vi "Create.vi"(8 "error in (no error)":errorcluster, 10 "Task Type":string) -> (0 "error out":errorcluster, 3 "TaskTypeIdentity out":refnum<class "TaskTypeIdentity.lvclass">)   [LabVIEW 2020, in "Volatus.lvlib" / "TaskTypeIdentity.lvclass"]
uses:
  TaskTypeIdentity.lvclass
  TaskTypeIdentity.lvclass/TaskTypeIdentity.ctl
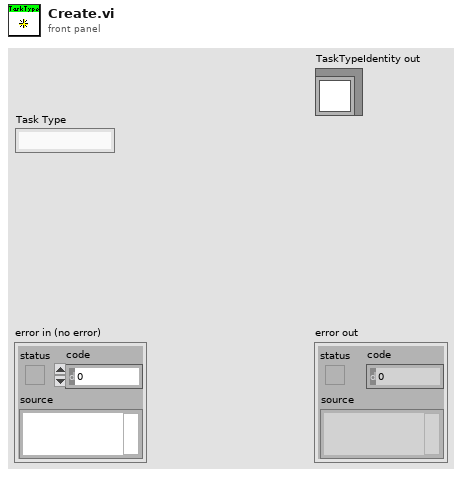
[diagram p1: front panel]
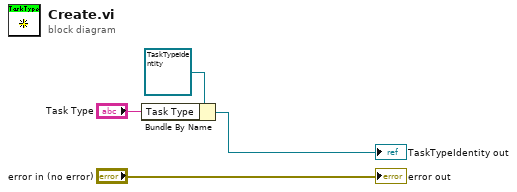
[diagram p0: block diagram]
diagram:
  n1 = Bundle By Name(cluster=refnum<class "TaskTypeIdentity.lvclass"> refnum ("TaskTypeIdentity in"), "Task Type"="Task Type") -> (→"TaskTypeIdentity out":refnum<class "TaskTypeIdentity.lvclass">)
  "error out" <- "error in (no error)"
